vi "语音数据.vi"(11 "path":path caption="路径") -> (3 "数组":dbl[](array[numeric]))   [LabVIEW 2018]
panel:
  out "波形图":waveform(dbl)[](graph)
  out "error out":errorcluster caption="错误输出"
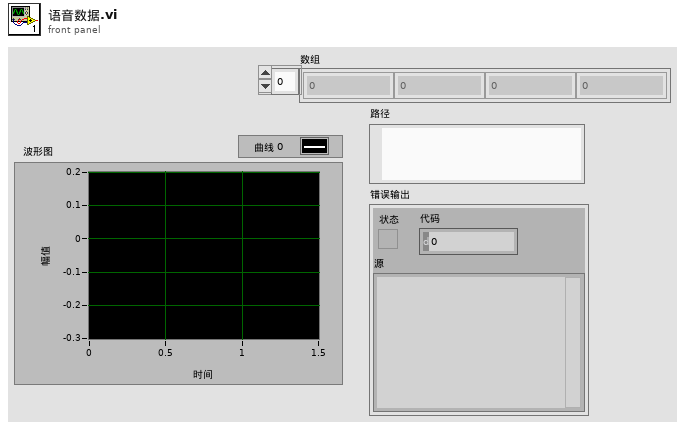
[diagram p1: front panel]
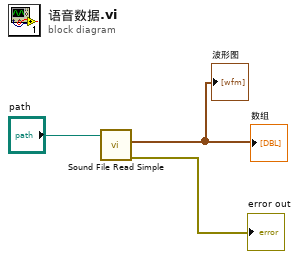
[diagram p0: block diagram]
diagram:
  n1 = call <vilib>:"Sound File Read Simple.vi"("path"="path") -> ("error out"=→"error out":errorcluster, "data"=→"数组" →"波形图":waveform(dbl)[])  [unwired: 7 in, 2 out]
